vi "Configure aver times.vi"(8 "error in (no error)":errorcluster, 9 "Trace":u16(ring) items=["Trace A", "Trace B", "Trace C", "Trace D", "Trace E"], 10 "Averaging times":i32=1, 11 "VISA resource name":refnum<visa-resource-name>) -> (0 "error out":errorcluster, 3 "VISA resource name out":refnum<visa-resource-name>)   [LabVIEW 2021, in "Ceyear.lvlib"]
uses:
  <instrlib>/Ceyear/Ceyear.lvlib
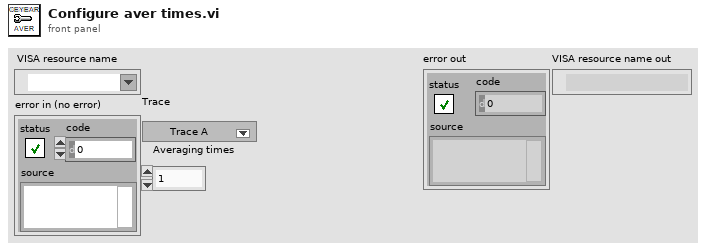
[diagram p1: front panel]
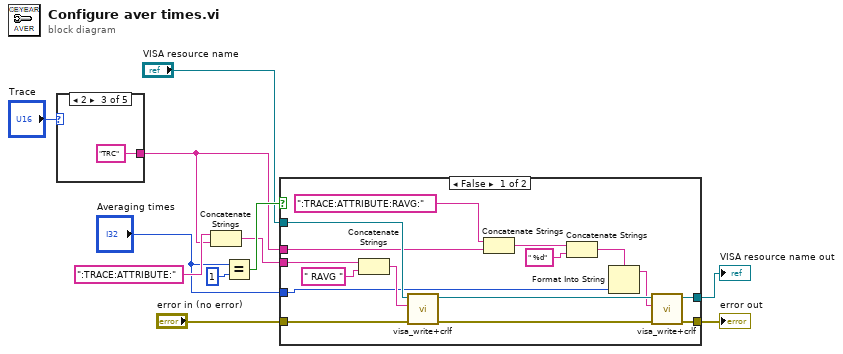
[diagram p0: block diagram]
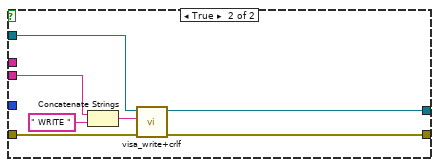
[diagram p2: hidden frame]
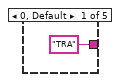
[diagram p3: hidden frame]
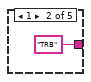
[diagram p4: hidden frame]
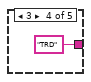
[diagram p5: hidden frame]
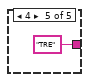
[diagram p6: hidden frame]
diagram:
  n1 = case shown="2" "Trace" {
    tunnel: ["TRA" "TRB" "TRC" "TRD" "TRE"] -> w2
    frame 0, Default {
    }
    frame 1 {
    }
    frame 2 {
    }
    frame 3 {
    }
    frame 4 {
    }
  }
  n2 = Concatenate Strings(":TRACE:ATTRIBUTE:", w2) -> (w8:string)
  n3 = Equal?(x="Averaging times", y=1) -> (x = y?=w9:bool)
  n4 = case shown="False" w9 {
    tunnel: w8 -> [w32 w38]
    tunnel: "VISA resource name" -> [w28 w37]
    tunnel: "error in (no error)" -> [w27 w36]
    tunnel: [w21 w34] -> w5
    tunnel: [w20 w33] -> w4
    tunnel: w2 -> [w24 _]
    tunnel: "Averaging times" -> [w19 _]
    frame False {
      n5 = Concatenate Strings(w32, " RAVG ") -> (w29:string)
      n6 = call <instrlib>:"visa_write+crlf.vi"("error in (no error)"=w27, "Strings (empty)"=w29, "VISA resource name"=w28) -> ("error out"=w30:errorcluster, "VISA resource name out"=w31:refnum<visa-resource-name>)  [unwired: 7 in]
      n7 = Concatenate Strings(":TRACE:ATTRIBUTE:RAVG:", w24) -> (w23:string)
      n8 = Concatenate Strings(w23, " %d" ("string")) -> (w18:string)
      n9 = Format Into String(format string=w18, w19) -> (resulting string=w17:string)  [unwired: 2 in, 1 out]
      n10 = call <instrlib>:"visa_write+crlf.vi"("error in (no error)"=w30, "Strings (empty)"=w17, "VISA resource name"=w31) -> ("error out"=w20:errorcluster, "VISA resource name out"=w21:refnum<visa-resource-name>)  [unwired: 7 in]
    }
    frame True {
      n11 = Concatenate Strings(w38, " WRITE ") -> (w35:string)
      n12 = call <instrlib>:"visa_write+crlf.vi"("error in (no error)"=w36, "Strings (empty)"=w35, "VISA resource name"=w37) -> ("error out"=w33:errorcluster, "VISA resource name out"=w34:refnum<visa-resource-name>)  [unwired: 7 in]
    }
  }
  "error out" <- w4
  "VISA resource name out" <- w5
